vi "Fs (Hz) Write.vi"(4 "error in (no error)":errorcluster, 5 "Value":dbl, 6 "Container State":T2, 7 "Display State In":T1={"Update"=FALSE, "Show advanced"=FALSE, "Fs (Hz)"=100000.0, "Show persist"=FALSE}) -> (0 "error out":errorcluster, 3 "Display State Out":T1={"Update"=FALSE, "Show advanced"=FALSE, "Fs (Hz)"=100000.0, "Show persist"=FALSE})   [LabVIEW 2020, in "Stimulus Channel (Full).xctl"]
uses:
  Stimulus Channel (Full).xctl
  <vilib>/_xctls/Container State.ctl
  State.ctl
  <vilib>/_xctls/XControlSupport.lvlib
panel:
  # "Replace the Value Control below with a Control of desired type.\nDo not remove this Control or the others from the connector pane.\nDo not change the connector pane pattern.\nThe Value control should always be the third terminal from top on the input side in the connector pane."
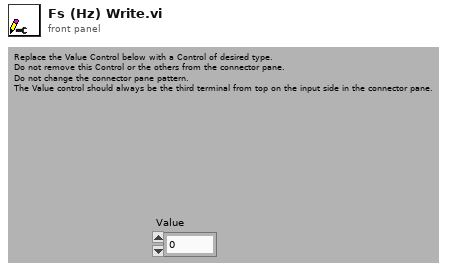
[diagram p1: front panel]
types:
  T1 = typedef "Stimulus Channel (Full).xctl/State.ctl" = cluster{"Update":bool, "Show advanced":bool, "Fs (Hz)":dbl, "Show persist":bool}
  T2 = typedef "XControlSupport.lvlib/Container State.ctl" = cluster{"Indicator?":bool, "Run Mode?":bool, " Refnum":refnum<vi>}
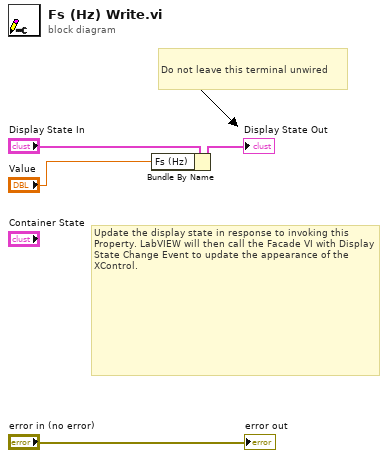
[diagram p0: block diagram]
diagram:
  # "Do not leave this terminal unwired"
  # "Update the display state in response to invoking this Property. LabVIEW will then call the Facade VI with Display State Change Event to update the appearance of the XControl."
  n1 = Bundle By Name(cluster="Display State In", "Fs (Hz)"="Value") -> (→"Display State Out":T1)
  "error out" <- "error in (no error)"
